vi "Manage Cycle Memory.vi"(6 "Operation":T1=enum."Write", 10 "Address":u32, 11 "Write Data":u64) -> (3 "Read Data":u64)   [LabVIEW 2017, in "FPGA-SRL.lvlib"]
uses:
  FPGA-SRL.lvlib
  user.lib/Utilities/Type Defs/MISC IO Choice Enum.ctl
  <vilib>/rvi/DataTransferAndStorage/Container/XNode/niFpgaContainer.xnode
  <vilib>/rvi/Memory/Memory_Emulation/nirvimemoryFastEmulation.vi
  <vilib>/rvi/Memory/Memory_Emulation/nirvimemoryEmulation.vi
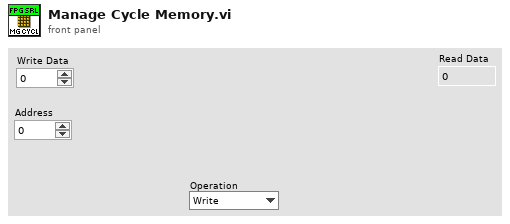
[diagram p1: front panel]
types:
  T1 = typedef "MISC IO Choice Enum.ctl" = enum16{"Read", "Write"}
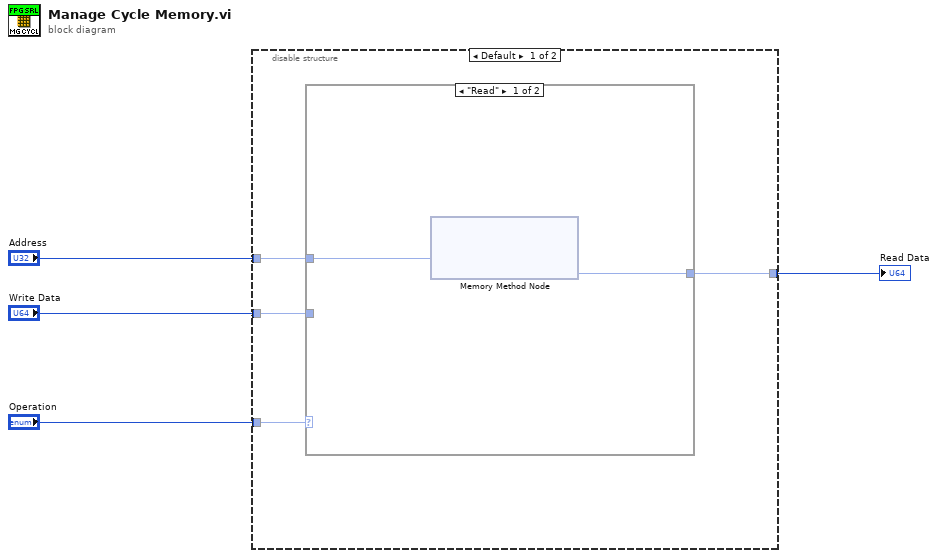
[diagram p0: block diagram]
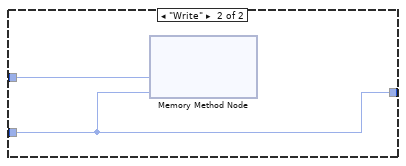
[diagram p2: hidden frame]
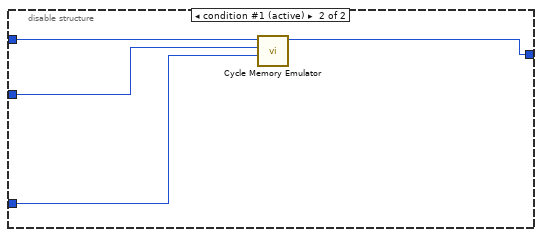
[diagram p3: hidden frame]
diagram:
  n1 = disable-structure shown="Default" {
    disable-tunnel: "Address" -> [w8 w16]
    disable-tunnel: "Write Data" -> [w7 w15]
    disable-tunnel: "Operation" -> [w6 w14]
    disable-tunnel: [w5 w13] -> w1
    frame condition #0 {
      n2 = case shown="\"Read\"" w6 {
        tunnel: w8 -> [w10 w12]
        tunnel: w7 -> [_ w11]
        tunnel: [w9 w11] -> w5
        frame "Read" {
          n3 = xnode ("Memory Method Node")("Address"=w10) -> ("Data"=w9:u64)  [unwired: 1 in, 1 out]
        }
        frame "Write" {
          n4 = xnode ("Memory Method Node")("Address"=w12, "Data"=w11) -> ()  [unwired: 1 in, 1 out]
        }
      }
    }
    frame condition #1 (active) {
      n5 = call "Cycle Memory Emulator.vi"("Operation"=w14, "Write Data in"=w15, "Address"=w16) -> ("Write Data out"=w13:u64)  [unwired: 8 in]
    }
  }
  "Read Data" <- w1
